vi "Get Trigger Pulse Width Ns Max.vi"(8 "error in (no error)":errorcluster) -> (0 "error out":errorcluster, 3 "function return":i32)   [LabVIEW 2021, in "vmmso.lvlib"]
doc: "DLL_API int WINAPI GetTriggerPulseWidthNsMax();"
uses:
  vmmso.lvlib
  vmmso.dll
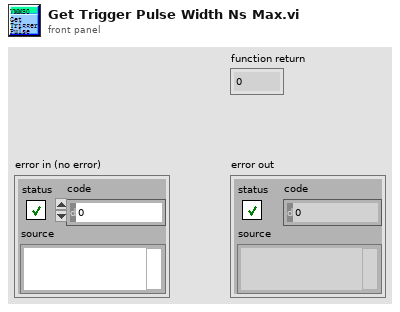
[diagram p1: front panel]
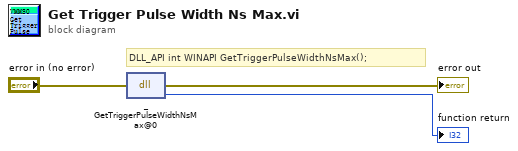
[diagram p0: block diagram]
diagram:
  # "DLL_API int WINAPI GetTriggerPulseWidthNsMax();"
  n1 = dll-call lib="O:/MSO/library/demo-Labview/vmmso/vmmso.*" fn="_GetTriggerPulseWidthNsMax@0"(error in="error in (no error)") -> (error out=→"error out":errorcluster, →"function return":i32)  [unwired: 2 in, 1 out]
